vi "SetRampMode.vi"(8 "error in (no error)":errorcluster, 11 "Laser Diode Controller in":refnum<class "KLD101.lvclass">) -> (0 "error out":errorcluster, 3 "Laser Diode Controller out":refnum<class "KLD101.lvclass">)   [LabVIEW 2016, in "Laser Diode Controller.lvlib" / "KLD101.lvclass"]
uses:
  KLD101.lvclass
  KLD101.lvclass/KLD101.ctl
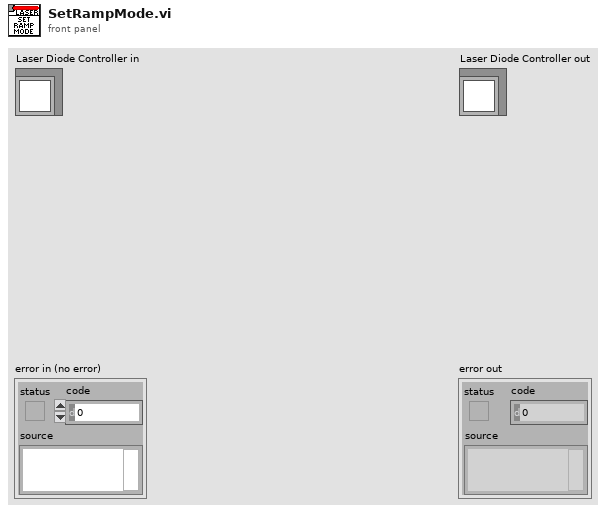
[diagram p1: front panel]
types:
  T1 = typedef "Configuration.lvlib/Config Data.lvclass/LaserRampMode.ctl" = enum16{"Immediate", "Ramped"}
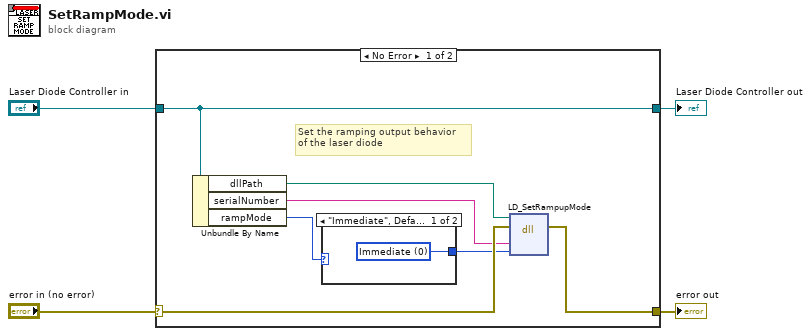
[diagram p0: block diagram]
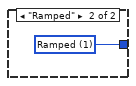
[diagram p2: hidden frame]
diagram:
  n1 = case shown="No Error" "error in (no error)" {
    selector: "error in (no error)" -> [w9 w15]
    tunnel: [w7 w15] -> w3
    tunnel: [w11 w14] -> w1
    tunnel: "Laser Diode Controller in" -> [w11 w14]
    frame No Error {
      # "Set the ramping output behavior\nof the laser diode"
      n2 = Unbundle By Name(w11) -> ("dllPath"=w5:path, "serialNumber"=w6:string, "rampMode"=w10:T1)
      n3 = case shown="\"Immediate\", Default" w10 {
        tunnel: [w12 w13] -> w8
        frame "Immediate", Default {
          w12 = u16 0 items=["Immediate", "Ramped"] ("rampUpMode")
        }
        frame "Ramped" {
          w13 = u16 1 items=["Immediate", "Ramped"] ("rampUpMode")
        }
      }
      n4 = dll-call lib="C:/IDEXX Software/Collimation/data/Thorlabs.MotionControl.KCube.LaserDiode.dll" fn="LD_SetRampupMode"(path in=w5, error in=w9, "serialNumber"=w6, "rampupMode"=w8) -> (error out=w7:errorcluster)  [unwired: 4 in, 1 out]
    }
    frame Error {
    }
  }
  "error out" <- w3
  "Laser Diode Controller out" <- w1
